vi "LVtest16.vi"() -> ()   [LabVIEW 2016]
uses:
  <vilib>/Instr/_visa.llb/VISA Configure Serial Port (Instr).vi
  milGrabber/vs2017/x64/Debug/milGrabberInterface.dll
panel:
  out "Higher image":u16[][](graph)
  out "Lower image":u16[][](graph)
  in  "index (row) 2":i32
  out "frame size":i64
  in  "index (row)":i32
  out "get":i32
  out "error out 4":errorcluster
  out "read buffer":string
  out "error out 3":errorcluster
  out "error out 2":errorcluster
  out "error out":errorcluster
  out "Intensity Graph":u8[][](graph)
  out "destroy":i32
  out "Start":i32
  out "int":i32
  # "775 * 385 * 4 = 1193500"
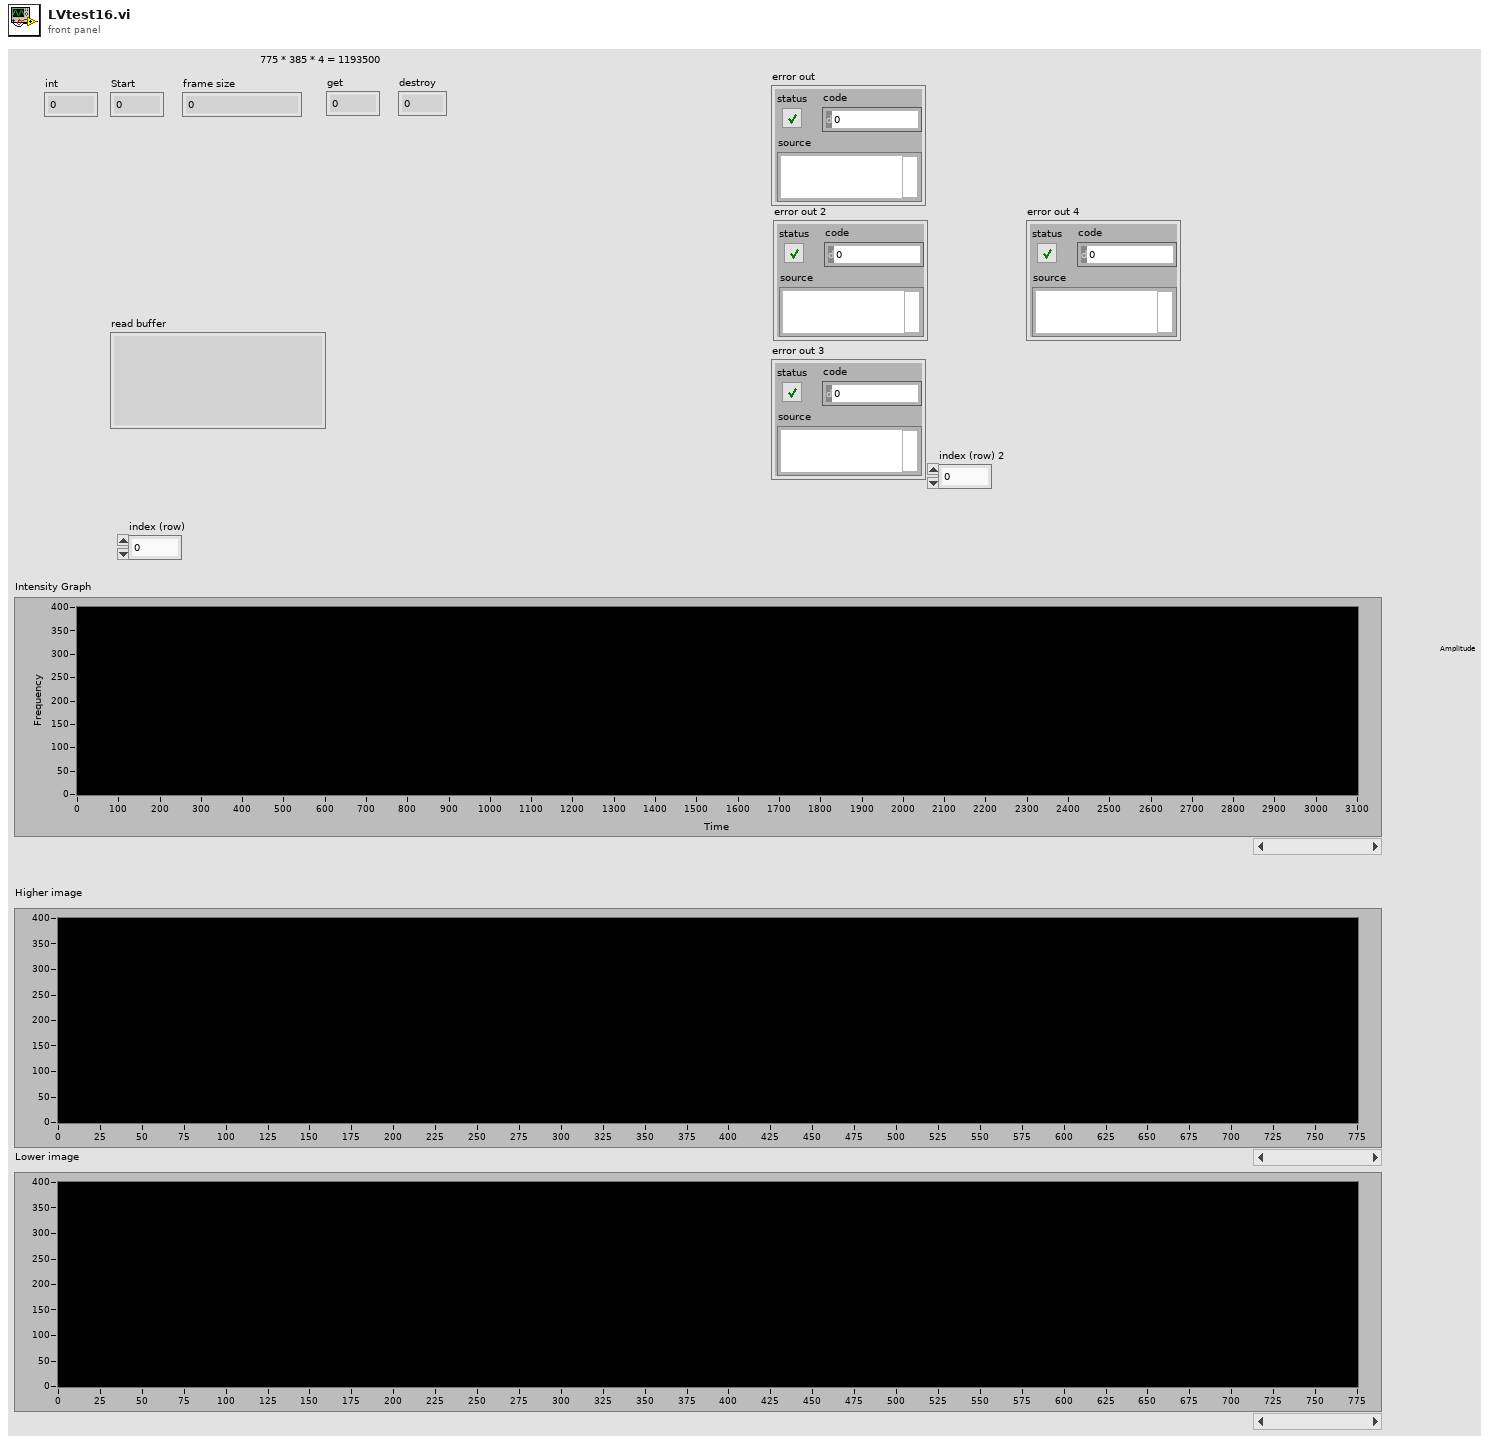
[diagram p1: front panel]
types:
  T1 = enum16{"big-endian, network order", "native, host order", "little-endian"}
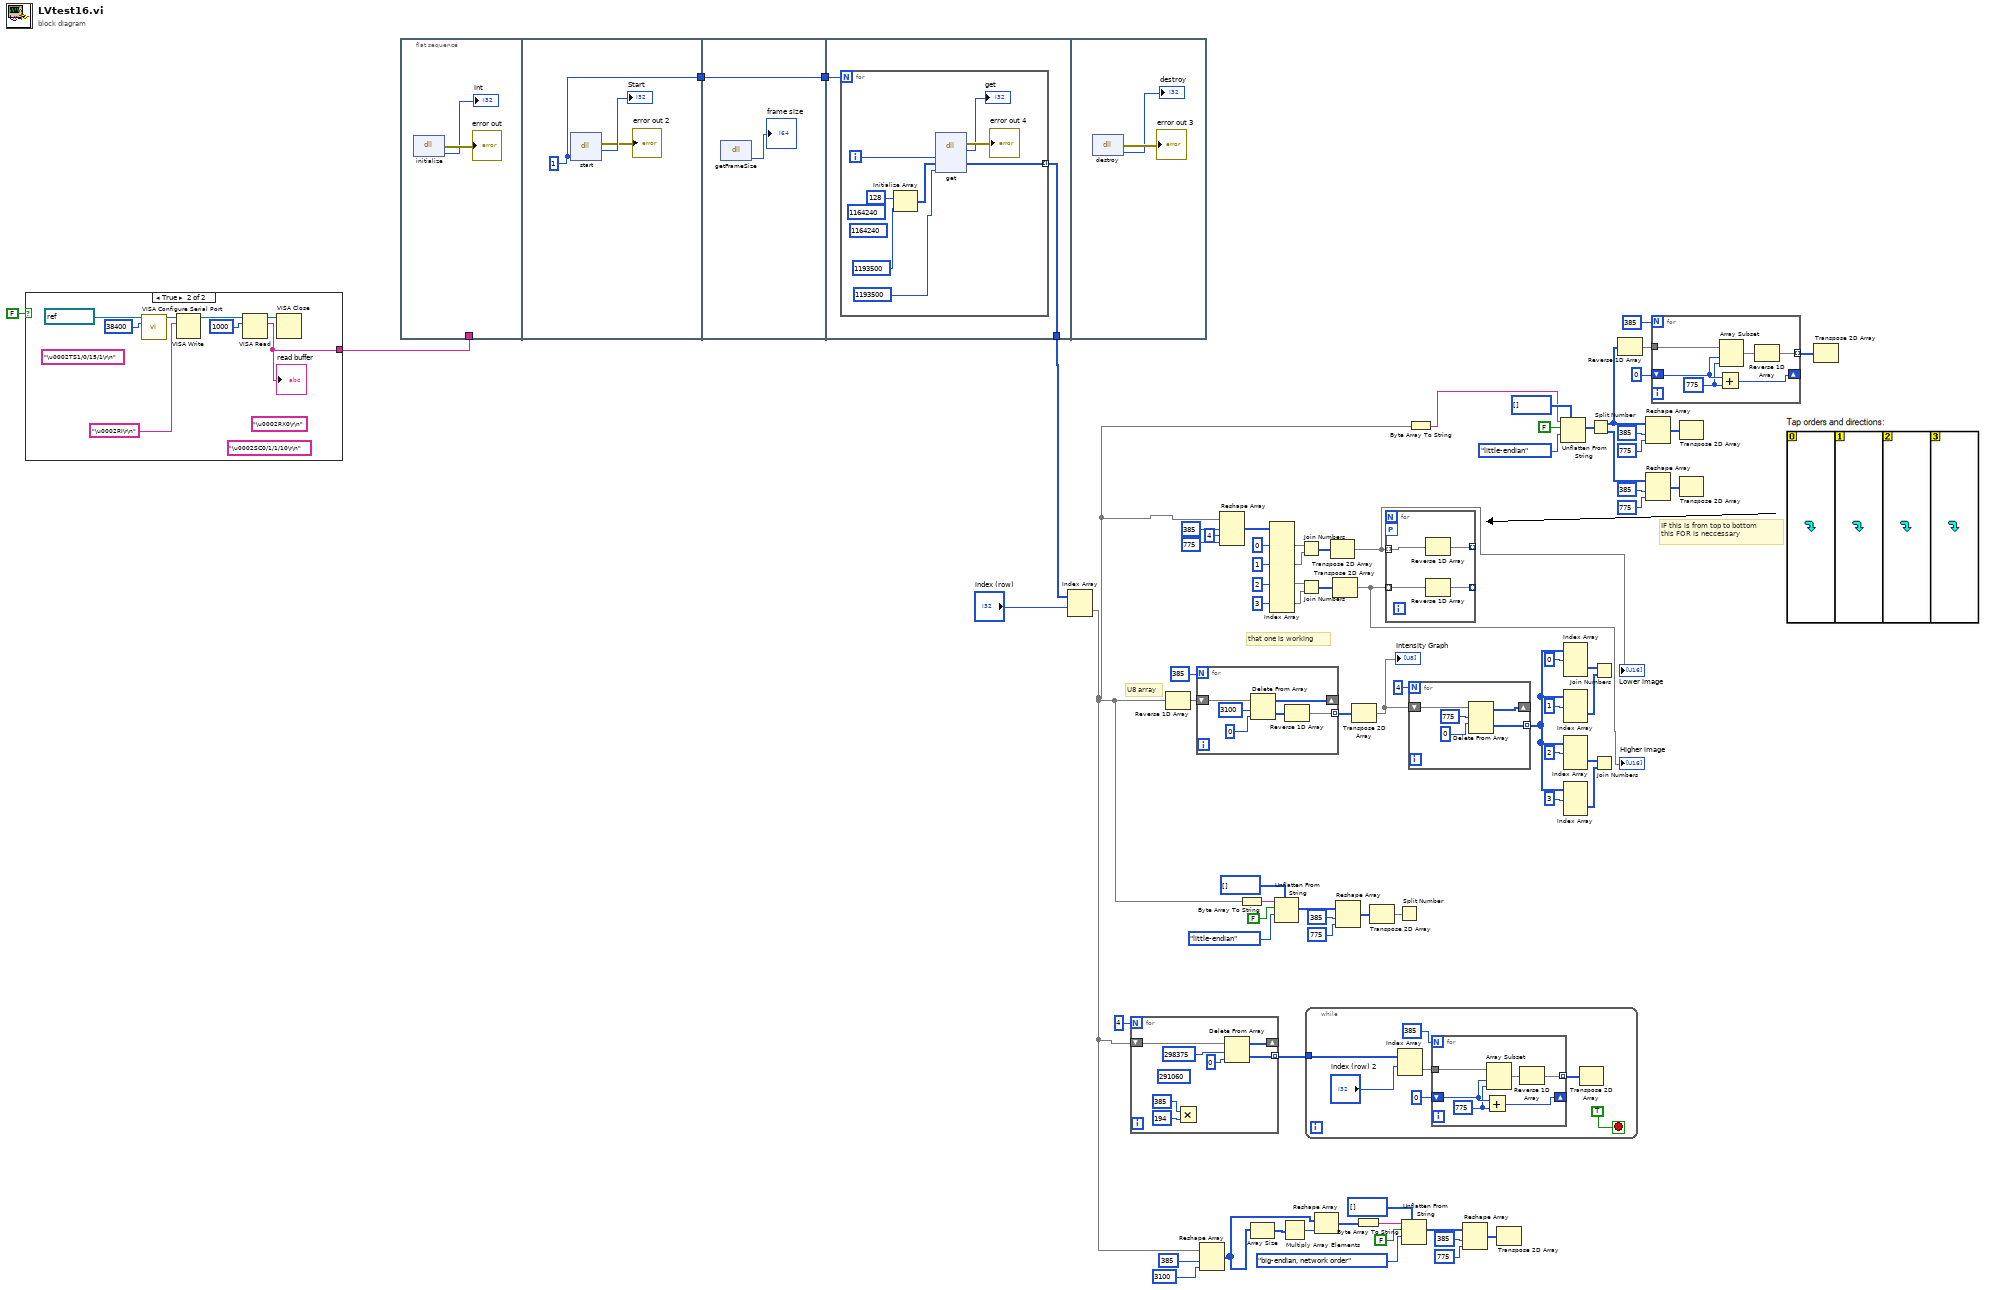
[diagram p0: block diagram]
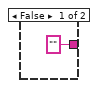
[diagram p2: hidden frame]
diagram:
  # "IF this is from top to bottom \nthis FOR is neccessary"
  # "U8 array"
  # "that one is working"
  n1 = case shown="True" FALSE {
    tunnel: ["" ("read buffer") w82] -> w78
    frame False {
    }
    frame True {
      (unwired) "\u0002SC0/1/1/10\r\n" ("format string")
      (unwired) "\u0002RX0\r\n" ("format string")
      (unwired) "\u0002TS1/0/15/1\r\n" ("format string")
      n2 = call-poly "VISA Configure Serial Port"("VISA resource name"=refnum<visa-resource-name> "COM3", "baud rate (9600)"=u32 38400) -> ("VISA resource name out"=w86:refnum<visa-resource-name>)  [unwired: 12 in, 1 out]
      n3 = VISA Write(VISA resource name=w86, write buffer="\u0002RI\r\n" ("format string")) -> (VISA resource name out=w85:refnum<visa-resource-name>)  [unwired: 1 in, 2 out]
      n4 = VISA Read(VISA resource name=w85, byte count=u32 1000) -> (VISA resource name out=w84:refnum<visa-resource-name>, read buffer=w82:string)  [unwired: 1 in, 2 out]
      "read buffer" <- w82
      n5 = VISA Close(VISA resource name=w84) -> ()  [unwired: 1 in, 1 out]
    }
  }
  n6 = flat-sequence {
    tunnel: [w89] -> _
    tunnel: w78 -> [w89]
    tunnel: [w92] -> w76
    tunnel: w76 -> [w96]
    tunnel: [w96] -> w75
    tunnel: w75 -> [w98]
    tunnel: [w97] -> w77
    frame #0 {
      n7 = dll-call lib="C:/Users/Kinga/Desktop/Matrox/Testy/milGrabber/vs2017/x64/Debug/milGrabberInterface.dll" fn="initialize"() -> (error out=→"error out":errorcluster, "int"=→"int":i32)  [unwired: 3 in, 1 out]
    }
    frame #1 {
      w92 = i16 1 ("grabFramesNo")
      n8 = dll-call lib="C:/Users/Kinga/Desktop/Matrox/Testy/milGrabber/vs2017/x64/Debug/milGrabberInterface.dll" fn="start"("grabFramesNo"=w92) -> (error out=→"error out 2":errorcluster, "int"=→"Start":i32)  [unwired: 4 in, 1 out]
    }
    frame #2 {
      n9 = dll-call lib="C:/Users/Kinga/Desktop/Matrox/Testy/milGrabber/vs2017/x64/Debug/milGrabberInterface.dll" fn="getFrameSize"() -> ("int"=→"frame size":i64)  [unwired: 3 in, 2 out]
    }
    frame #3 {
      n10 = for {
        N: w98 -> [_]
        tunnel: [w101] -> w97 mode=indexing
        i -> [w102]
        (unwired) 1164240 ("out_size")
        (unwired) 1164240 ("dimension size")
        n11 = Initialize Array(u8 128 ("element"), 1193500 ("out_size")) -> (w103:u8[])
        n12 = dll-call lib="C:/Users/Kinga/Desktop/Matrox/Testy/milGrabber/vs2017/x64/Debug/milGrabberInterface.dll" fn="get"("frameNum"=w102, "out_buf"=w103, "out_size"=1193500 ("dimension size")) -> (error out=→"error out 4":errorcluster, "int"=→"get":i32, "out_buf"=w101:u8[])  [unwired: 5 in, 1 out]
      }
    }
    frame #4 {
      n13 = dll-call lib="C:/Users/Kinga/Desktop/Matrox/Testy/milGrabber/vs2017/x64/Debug/milGrabberInterface.dll" fn="destroy"() -> (error out=→"error out 3":errorcluster, "int"=→"destroy":i32)  [unwired: 3 in, 1 out]
    }
  }
  n14 = Index Array(array=w77, index (row)="index (row)") -> (element=w3:u8[])  [unwired: 1 in]
  n15 = for {
    N: 4 -> [_]
    shift-right: [w115] -> _
    shift-left: w3 -> [w110]
    tunnel: [w111] -> w43 mode=indexing
    (unwired) 291060 ("length")
    n16 = Multiply(x=385, y=194 ("length")) -> ()  [unwired: 1 out]
    n17 = Delete From Array(array=w110, length=298375, index=0) -> (deleted portion=w111:u8[], array with subset deleted=w115:u8[])
  }
  n18 = Reverse 1D Array(array=w3) -> (reversed array=w30:u8[])
  n19 = for {
    N: 385 -> [_]
    tunnel: [w121] -> w31 mode=indexing
    shift-right: [w118] -> _
    shift-left: w30 -> [w119]
    n20 = Delete From Array(array=w119, length=3100, index=0) -> (deleted portion=w120:u8[], array with subset deleted=w118:u8[])
    n21 = Reverse 1D Array(array=w120) -> (reversed array=w121:u8[])
  }
  n22 = Reshape Array(w3, 385 ("dimension size"), 3100 ("dimension size")) -> (w44:u8[][])
  n23 = Reshape Array(w3, 385, 4 ("dimension size"), 775 ("length")) -> (w5:u8[][][])
  n24 = Byte Array To String(unsigned byte array=w3) -> (string=w50:string)
  n25 = Array Size(array=w44) -> (size(s)=w70:i32[])
  n26 = Index Array(array=w5, index (dim 1) #1=0 ("disabled index (row)"), index (dim 1) #2=1 ("index (row)"), index (dim 1) #3=2 ("disabled index (row)"), index (dim 1) #4=3 ("index (row)")) -> (element #1=w16:u8[][], element #2=w11:u8[][], element #3=w10:u8[][], element #4=w9:u8[][])  [unwired: 8 in]
  n27 = Unflatten From String(type=u32[] [] ("U32 Array"), binary string=w50, data includes array or string size? (T)=FALSE, byte order (0:big-endian, network order)=T1."little-endian") -> (value=w45:u32[])  [unwired: 1 in, 2 out]
  n28 = Multiply Array Elements(1:w70) -> (0:w71:i32)
  n29 = Join Numbers(hi=w16, lo=w11) -> ((hi.lo)=w4:u16[][])
  n30 = Join Numbers(hi=w10, lo=w9) -> ((hi.lo)=w8:u16[][])
  n31 = while {
    tunnel: w43 -> [w128]
    stop <- TRUE stop-if-true
    n32 = Index Array(array=w128, index (row)="index (row) 2") -> (element=w124:u8[])  [unwired: 1 in]
    n33 = for {
      N: 385 -> [_]
      tunnel: w124 -> [w133]
      tunnel: [w134] -> w123 mode=indexing
      shift-right: [w130] -> _
      shift-left: 0 -> [w131]
      w129 = 775 ("length")
      n34 = Add(x=w131, y=w129) -> (x+y=w130:i32)
      n35 = Array Subset(array=w133, index=w131, length=w129) -> (w132:u8[])
      n36 = Reverse 1D Array(array=w132) -> (reversed array=w134:u8[])
    }
    n37 = Transpose 2D Array(2D array=w123) -> ()  [unwired: 1 out]
  }
  n38 = Reshape Array(w44, w71) -> (w69:u8[])
  n39 = Transpose 2D Array(2D array=w4) -> (transposed array=w1:u16[][])
  "Lower image" <- w1
  n40 = Transpose 2D Array(2D array=w8) -> (transposed array=w2:u16[][])
  "Higher image" <- w2
  n41 = Reshape Array(w45, 385 ("dimension size"), 775 ("dimension size")) -> (w47:u32[][])
  n42 = Transpose 2D Array(2D array=w31) -> (transposed array=w27:u8[][])
  "Intensity Graph" <- w27
  n43 = Byte Array To String(unsigned byte array=w69) -> (string=w68:string)
  n44 = Transpose 2D Array(2D array=w47) -> (transposed array=w41:u32[][])
  n45 = for {
    tunnel: w1 -> [w138] mode=indexing
    tunnel: [w137] -> _ mode=indexing
    tunnel: w2 -> [w136] mode=indexing
    tunnel: [w135] -> _ mode=indexing
    workers-P: _ -> [_]
    n46 = Reverse 1D Array(array=w138) -> (reversed array=w137:u16[])
    n47 = Reverse 1D Array(array=w136) -> (reversed array=w135:u16[])
  }
  n48 = Split Number(x=w41) -> ()  [unwired: 2 out]
  n49 = Unflatten From String(type=u32[] [] ("U32 Array"), binary string=w68, data includes array or string size? (T)=FALSE, byte order (0:big-endian, network order)=T1."big-endian, network order") -> (value=w61:u32[])  [unwired: 1 in, 2 out]
  n50 = Byte Array To String(unsigned byte array=w3) -> (string=w59:string)
  n51 = for {
    N: 4 -> [_]
    shift-right: [w143] -> _
    shift-left: w27 -> [w141]
    tunnel: [w142] -> w20 mode=indexing
    n52 = Delete From Array(array=w141, length=775, index (row)=0) -> (deleted portion=w142:u8[][], array with subset deleted=w143:u8[][])  [unwired: 1 in]
  }
  n53 = Reshape Array(w61, 385 ("dimension size"), 775 ("dimension size")) -> (w62:u32[][])
  n54 = Transpose 2D Array(2D array=w62) -> ()  [unwired: 1 out]
  n55 = Unflatten From String(type=u32[] [] ("U32 Array"), binary string=w59, data includes array or string size? (T)=FALSE, byte order (0:big-endian, network order)=T1."little-endian") -> (value=w40:u32[])  [unwired: 1 in, 2 out]
  n56 = Index Array(array=w20, index (dim 0)=0 ("index (page)")) -> (element=w24:u8[][])  [unwired: 2 in]
  n57 = Index Array(array=w20, index (dim 0)=1 ("index (page)")) -> (element=w23:u8[][])  [unwired: 2 in]
  n58 = Index Array(array=w20, index (dim 0)=2 ("index (page)")) -> (element=w21:u8[][])  [unwired: 2 in]
  n59 = Index Array(array=w20, index (dim 0)=3 ("index (page)")) -> (element=w22:u8[][])  [unwired: 2 in]
  n60 = Split Number(x=w40) -> (hi(x)=w33:u16[], lo(x)=w42:u16[])
  n61 = Join Numbers(hi=w24, lo=w23) -> ()  [unwired: 1 out]
  n62 = Join Numbers(hi=w21, lo=w22) -> ()  [unwired: 1 out]
  n63 = Reverse 1D Array(array=w33) -> (reversed array=w29:u16[])
  n64 = Reshape Array(w33, 385 ("dimension size"), 775 ("dimension size")) -> (w39:u16[][])
  n65 = Reshape Array(w42, 385 ("dimension size"), 775 ("dimension size")) -> (w46:u16[][])
  n66 = for {
    N: 385 -> [_]
    tunnel: w29 -> [w148]
    tunnel: [w149] -> w34 mode=indexing
    shift-right: [w145] -> _
    shift-left: 0 -> [w146]
    w144 = 775 ("length")
    n67 = Add(x=w146, y=w144) -> (x+y=w145:i32)
    n68 = Array Subset(array=w148, index=w146, length=w144) -> (w147:u16[])
    n69 = Reverse 1D Array(array=w147) -> (reversed array=w149:u16[])
  }
  n70 = Transpose 2D Array(2D array=w39) -> ()  [unwired: 1 out]
  n71 = Transpose 2D Array(2D array=w46) -> ()  [unwired: 1 out]
  n72 = Transpose 2D Array(2D array=w34) -> ()  [unwired: 1 out]
